vi "Items_get.vi"(8 "error in (no error)":errorcluster, 10 "Group":i32=1 min=1, 11 "OXY_SCPI Reseource In":refnum<visa-resource-name>) -> (0 "error out":errorcluster, 1 "communication_data":T1, 2 "Channels":string[](array[string]), 3 "OXY_SCPI Reseource Out":refnum<visa-resource-name>)   [LabVIEW 2020, in "OXYGEN_Datastream.lvlib"]
uses:
  OXYGEN_Datastream.lvlib
  TypeDefs/Cluster_RawCommData.ctl
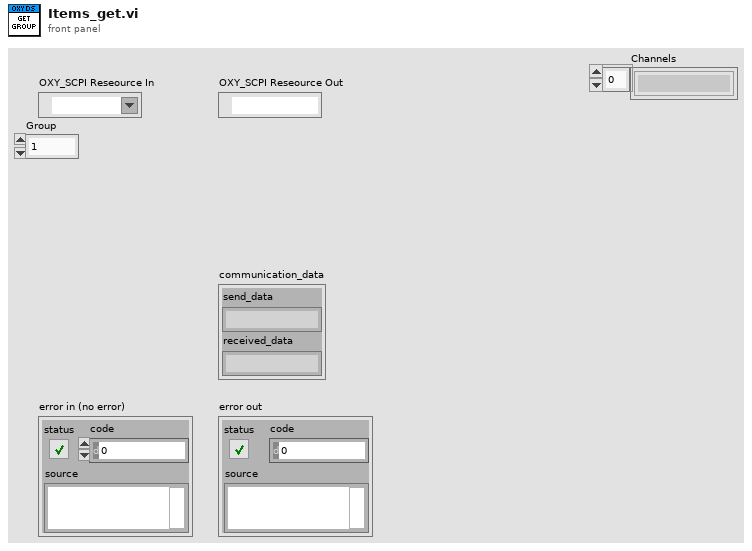
[diagram p1: front panel]
types:
  T1 = typedef "OXYGEN_Datastream.lvlib/Cluster_RawCommData.ctl" = cluster{"send_data":string, "received_data":string}
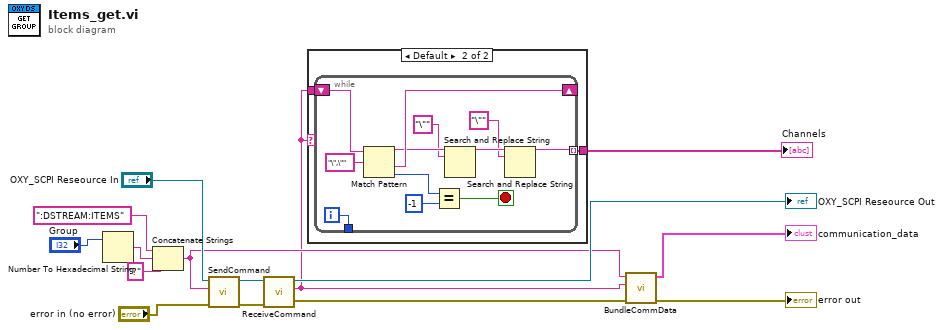
[diagram p0: block diagram]
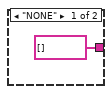
[diagram p2: hidden frame]
diagram:
  n1 = Number To Hexadecimal String(2:"Group") -> (0:w6:string)  [unwired: 1 in]
  n2 = Concatenate Strings(":DSTREAM:ITEMS", w6, "?" ("string")) -> (w5:string)
  n3 = call "SendCommand.vi"("error in (no error)"="error in (no error)", "String to Send"=w5, "OXY_SCPI Reseource In"="OXY_SCPI Reseource In") -> ("error out"=w15:errorcluster, "OXY_SCPI Reseource Out"=w14:refnum<visa-resource-name>)  [unwired: 7 in]
  n4 = call "ReceiveCommand.vi"("error in (no error)"=w15, "OXY_SCPI Reseource In"=w14) -> ("error out"=w13:errorcluster, "received Data"=w2:string, "OXY_SCPI Reseource Out"=→"OXY_SCPI Reseource Out":refnum<visa-resource-name>)  [unwired: 6 in, 1 out]
  n5 = case shown="Default" w2 {
    tunnel: [string[] [] w18] -> w4
    tunnel: w2 -> [_ w17]
    frame "NONE" {
    }
    frame Default {
      n6 = while {
        shift-right: [w25] -> _
        shift-left: w17 -> [w27]
        tunnel: [w21] -> w18 mode=indexing
        tunnel: [w19] -> _
        i -> [w19]
        stop <- w28 stop-if-true
        n7 = Match Pattern(string=w27, regular expression="\",\"") -> (before substring=w24:string, after substring=w25:string, offset past match=w30:i32)  [unwired: 1 in, 1 out]
        n8 = Equal?(x=w30, y=-1) -> (x = y?=w28:bool)
        n9 = Search and Replace String(input string=w24, search string="\"" ("substring (\"\")")) -> (result string=w22:string)  [unwired: 6 in, 3 out]
        n10 = Search and Replace String(input string=w22, search string="\"" ("substring (\"\")")) -> (result string=w21:string)  [unwired: 6 in, 3 out]
      }
    }
  }
  "Channels" <- w4
  n11 = call "BundleCommData.vi"("error in (no error)"=w13, "received_data"=w2, "send_data"=w5) -> ("error out"=→"error out":errorcluster, "communication_data"=→"communication_data":T1)  [unwired: 7 in]
